vi "数据查询_仪器数据.vi"() -> ()   [LabVIEW 2016]
uses:
  <vilib>/Utility/miscctls.llb/LVRowAndColumnUnsignedTypeDef.ctl
  <vilib>/Utility/miscctls.llb/LVPointTypeDef.ctl
panel:
  in  "工作模式":string(combo)="全部数据"
  in  "查询":bool
  in  "结束日期":string="2020/01/01"
  in  "起始日期":string="2010/01/01"
  in  "组合框":string(combo)
  out "数据表":string[][](table)
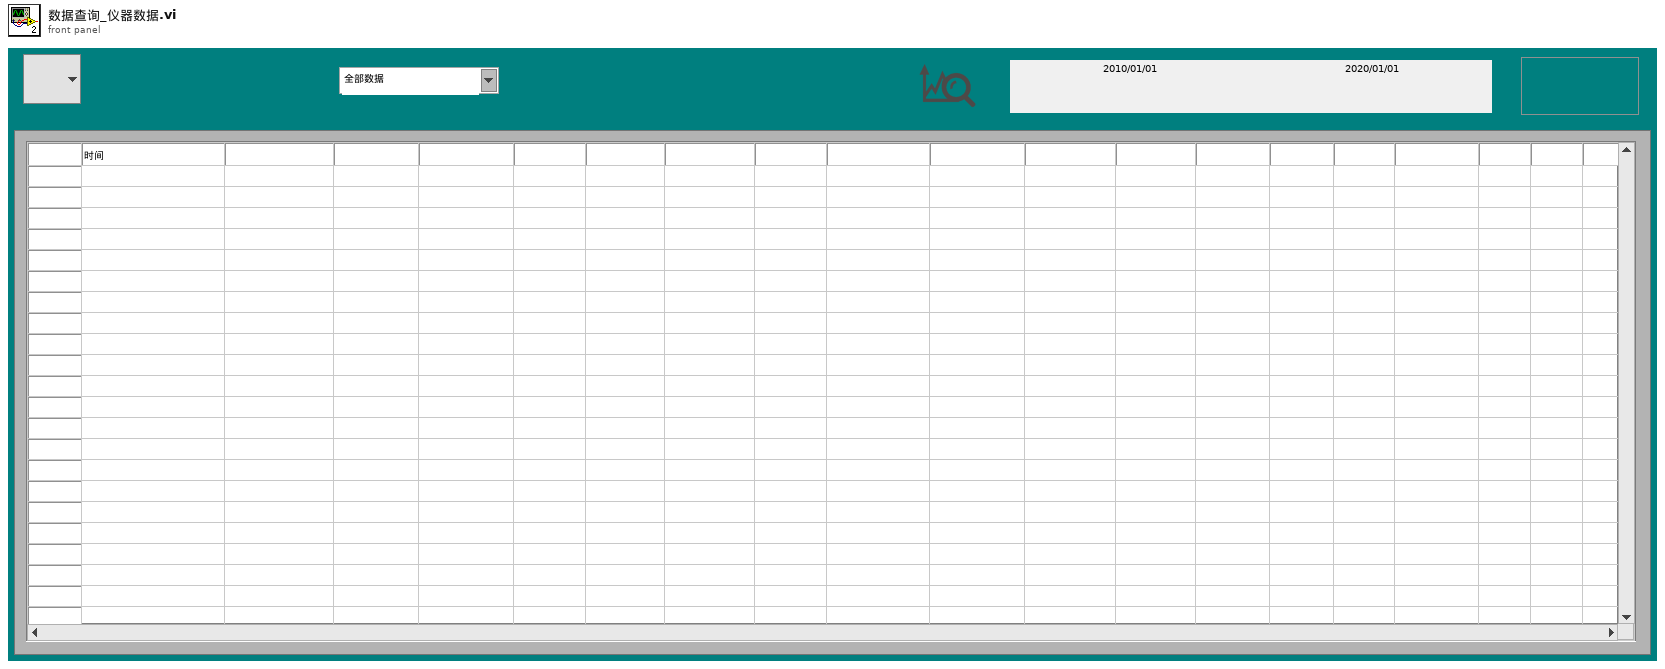
[diagram p1: front panel]
types:
  T1 = typedef "LVRowAndColumnUnsignedTypeDef.ctl" = cluster{"Row":u32, "Column":u32}
  T2 = typedef "LVPointTypeDef.ctl" = cluster{"Horizontal":i16, "Vertical":i16}
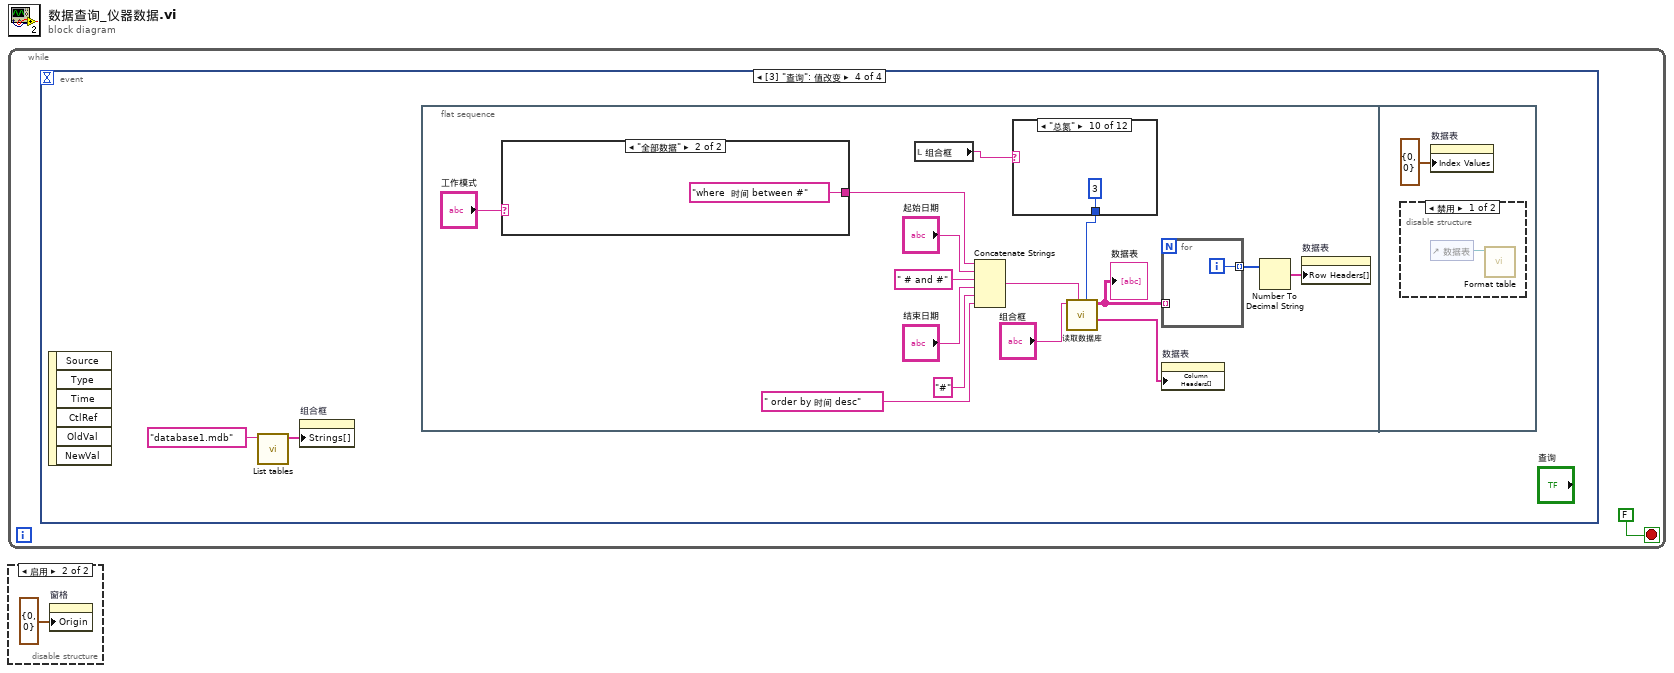
[diagram p0: block diagram]
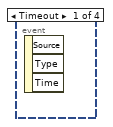
[diagram p2: hidden frame]
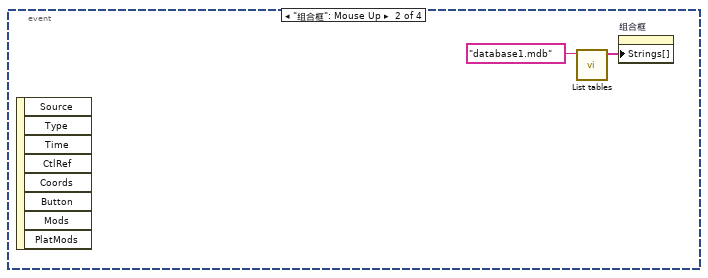
[diagram p3: hidden frame]
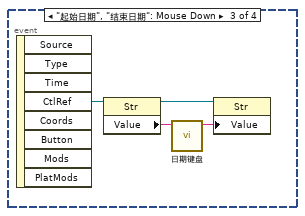
[diagram p4: hidden frame]
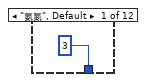
[diagram p5: hidden frame]
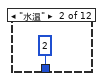
[diagram p6: hidden frame]
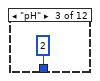
[diagram p7: hidden frame]
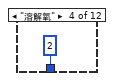
[diagram p8: hidden frame]
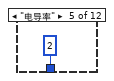
[diagram p9: hidden frame]
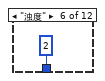
[diagram p10: hidden frame]
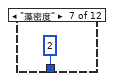
[diagram p11: hidden frame]
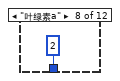
[diagram p12: hidden frame]
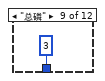
[diagram p13: hidden frame]
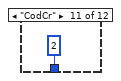
[diagram p14: hidden frame]
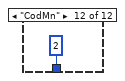
[diagram p15: hidden frame]
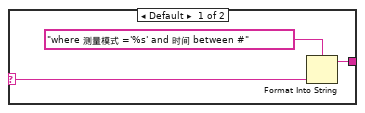
[diagram p16: hidden frame]
diagram:
  n1 = while {
    stop <- FALSE stop-if-true
    n2 = event shown="[3] \"查询\": 值改变" {
      selector: _ -> [_ _ _ _]
      dyn-events: _ -> [_ _ _ _]
      timeout: _ -> [_ _ _ _]
      event Timeout {
        n3 = event-data() -> ()  [unwired: 1 in, 3 out]
      }
      event "组合框": Mouse Up {
        n4 = event-data() -> ()  [unwired: 1 in, 8 out]
        n5 = call "List tables.vi"("database"="database1.mdb") -> ("tables"=w3:string[])  [unwired: 9 in, 1 out]
        n6 = property on="组合框" class="CmbBox"("Strings[]"=w3) -> ()  [unwired: 2 in, 2 out]
      }
      event "起始日期", "结束日期": Mouse Down {
        n7 = event-data() -> ("CtlRef"=w7:refnum<vi>)  [unwired: 1 in, 7 out]
        n8 = property class="Str"(reference=w7) -> (reference out=w5:refnum<vi>, "Value"=w6:string)  [unwired: 1 in, 1 out]
        n9 = call "日期键盘.vi"("原值"=w6) -> ("x+y"=w4:string)  [unwired: 10 in]
        n10 = property class="Str"(reference=w5, "Value"=w4) -> ()  [unwired: 1 in, 2 out]
      }
      event "查询": Value Change {
        n11 = event-data() -> ()  [unwired: 1 in, 6 out]
        n12 = call "List tables.vi"("database"="database1.mdb") -> ("tables"=w9:string[])  [unwired: 9 in, 1 out]
        n13 = property on="组合框" class="CmbBox"("Strings[]"=w9) -> ()  [unwired: 2 in, 2 out]
        n14 = flat-sequence {
          frame #0 {
            n15 = case shown="\"全部数据\"" "工作模式" {
              selector: "工作模式" -> [w39 _]
              tunnel: [w37 "where  时间 between #" ("condition")] -> w12
              frame Default {
                n16 = Format Into String(format string="where 测量模式 ='%s' and 时间 between #" ("condition"), w39) -> (resulting string=w37:string)  [unwired: 2 in, 1 out]
              }
              frame "全部数据" {
              }
            }
            n17 = local read "组合框"() -> (w11:string)
            n18 = Concatenate Strings(w12, "起始日期", " # and #" ("condition"), "结束日期", "#" ("condition"), " order by 时间 desc" ("字符串")) -> (w23:string)
            n19 = case shown="\"总氮\"" w11 {
              tunnel: [i16 3 ("精度(6)") i16 2 ("精度(6)") i16 2 ("精度(6)") i16 2 ("精度(6)") i16 2 ("精度(6)") i16 2 ("精度(6)") i16 2 ("精度(6)") i16 2 ("精度(6)") i16 3 ("精度(6)") i16 3 ("精度(6)") i16 2 ("精度(6)") i16 2 ("精度(6)")] -> w10
              frame "氨氮", Default {
              }
              frame "水温" {
              }
              frame "pH" {
              }
              frame "溶解氧" {
              }
              frame "电导率" {
              }
              frame "浊度" {
              }
              frame "藻密度" {
              }
              frame "叶绿素a" {
              }
              frame "总磷" {
              }
              frame "总氮" {
              }
              frame "CodCr" {
              }
              frame "CodMn" {
              }
            }
            n20 = call "读取数据库.vi"("精度(6)"=w10, "condition"=w23, "组合框"="组合框") -> ("columns"=w19:string[], "表格"=w16:string[][])  [unwired: 5 in, 2 out]
            "数据表" <- w16
            n21 = for {
              tunnel: w16 -> [_] mode=indexing
              tunnel: [w41] -> w15 mode=indexing
              i -> [w41]
            }
            n22 = property on="数据表" class="Tbl (严格)"("Column Headers[]"=w19) -> ()  [unwired: 2 in, 2 out]
            n23 = Number To Decimal String(number=w15) -> (decimal integer string=w14:string[])  [unwired: 1 in]
            n24 = property on="数据表" class="Tbl (严格)"("Row Headers[]"=w14) -> ()  [unwired: 2 in, 2 out]
          }
          frame #1 {
            n25 = disable-structure shown="禁用" {
              frame Disabled {
                n26 = control-ref of="数据表"() -> (w43:refnum<vi>)
                n27 = call "Format table.vi"("Table输入"=w43) -> ()  [unwired: 11 in]
              }
              frame Enabled {
              }
            }
            n28 = property on="数据表" class="Tbl (严格)"("Index Values"=T1 {"Row"=0, "Column"=0} ("索引值")) -> ()  [unwired: 2 in, 2 out]
          }
        }
      }
    }
  }
  n29 = disable-structure shown="启用" {
    frame Disabled {
    }
    frame Enabled {
      n30 = property on="窗格" class="Pane"("Origin"=T2 {"Horizontal"=0, "Vertical"=0} ("原点")) -> ()  [unwired: 2 in, 2 out]
    }
  }
